vi "tcp client example.vi"() -> ()   [LabVIEW 2013]
doc: "# #############################################################################\n# ATTENTION\n# #############################################################################\n#\n# This software is for guidance only. It is provided \"as is\".\n# It only aims at providing coding information to the customer in order for\n# them to save time. As a result no warranties, whether express, implied or\n# statutory, including, but not limited to implied warranties of\n# merchantability and fitness for a particular purpose apply to this software.\n# A·P·E Angewandte Physik und Elektronik GmbH shall not be held liable for any\n# direct, indirect or consequential damages with respect to any claims arising\n# from the content of such sourcecode and/or the use made by customers of the\n# coding information contained herein in connection with their products.\n#\n# #############################################################################"
uses:
  queue control/queue cluster.ctl
  <vilib>/Utility/miscctls.llb/LVPointTypeDef.ctl
panel:
  out "STOP":bool=TRUE
  out "error out":errorcluster
  out "Answer":string
  in  "Send":bool
  in  "CMD":string="*idn?\n" caption="Command"
  in  "Connect":bool
  in  "IP":string="127.0.0.1" caption="IP / Hostname"
  in  "PORT":u16=51019 caption="TCP Port"
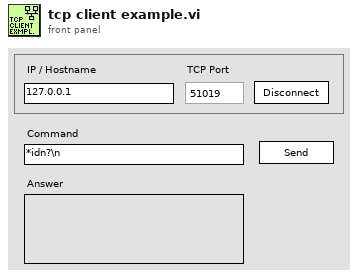
[diagram p1: front panel]
types:
  T1 = typedef "queue cluster.ctl" = cluster{"command":string, "data":variant}
  T2 = typedef "LVPointTypeDef.ctl" = cluster{"Horizontal":i16, "Vertical":i16}
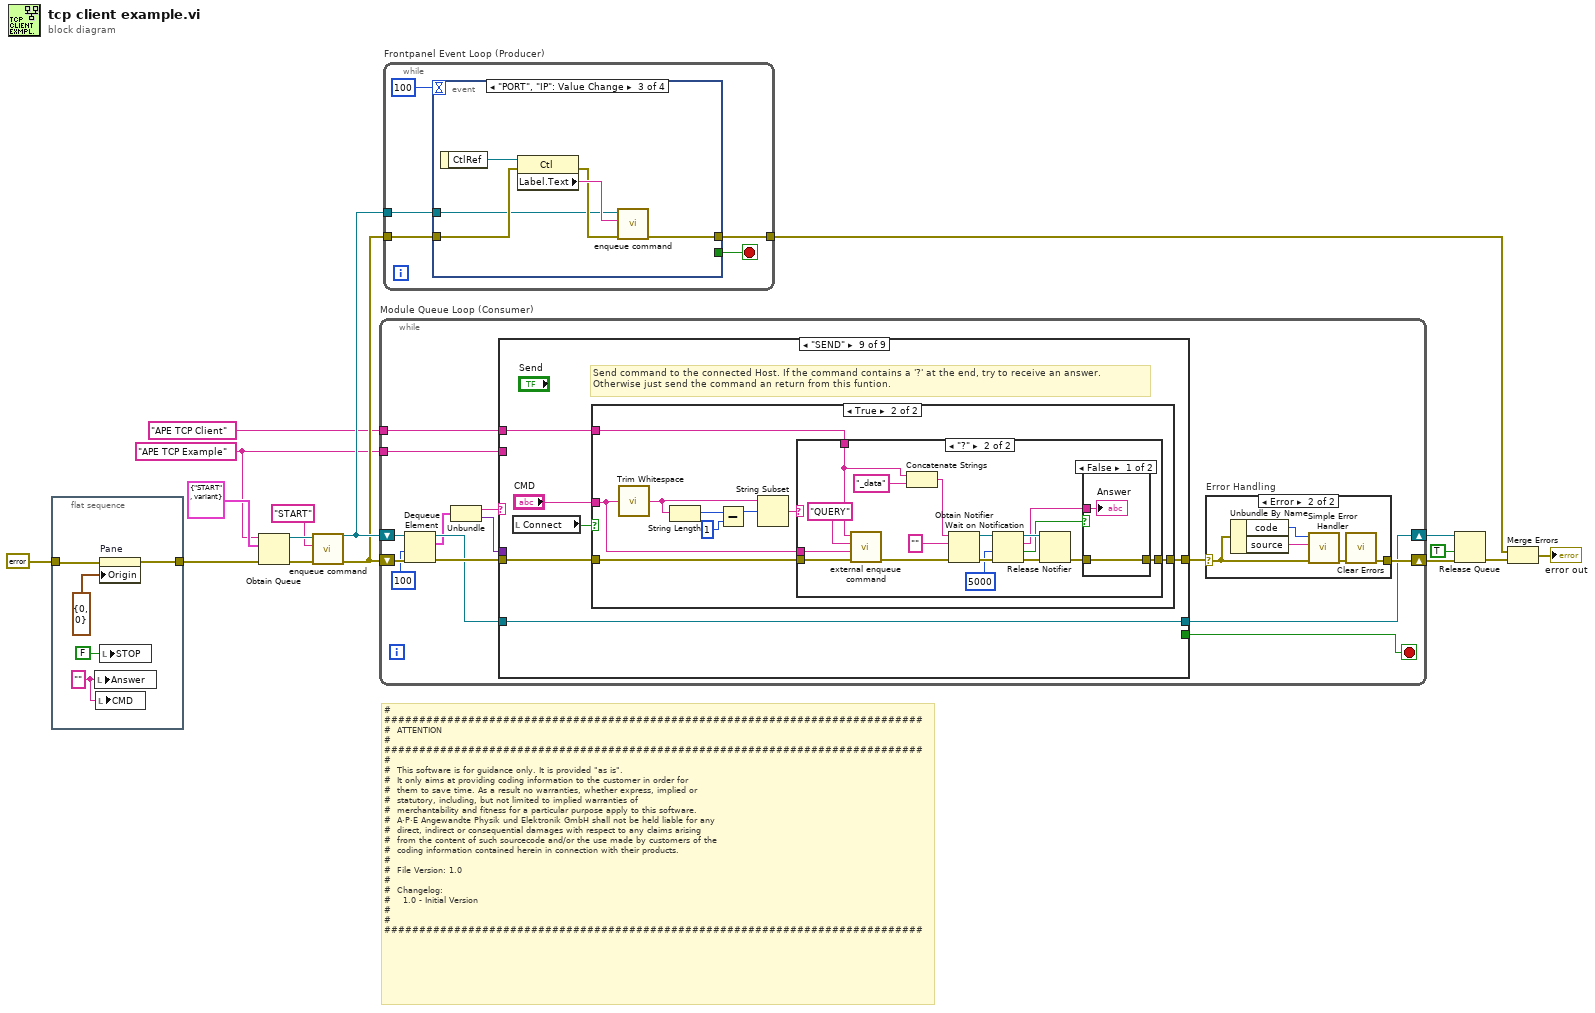
[diagram p0: block diagram]
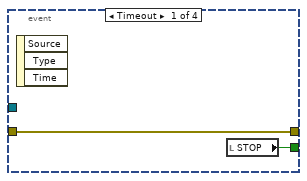
[diagram p2: hidden frame]
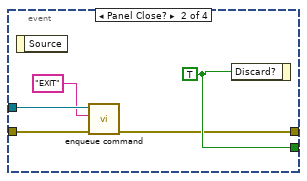
[diagram p3: hidden frame]
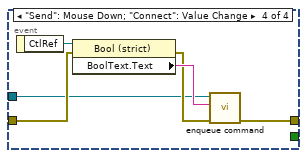
[diagram p4: hidden frame]
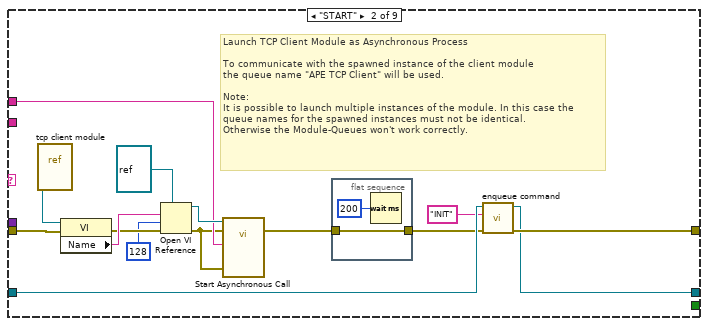
[diagram p7: hidden frame]
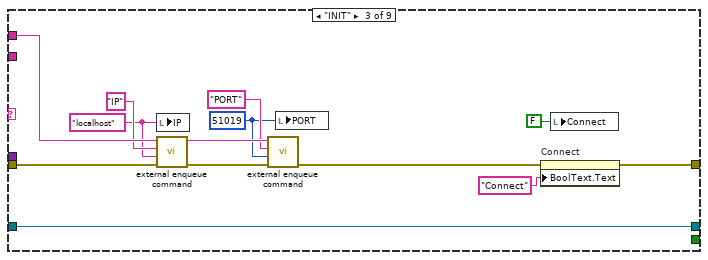
[diagram p8: hidden frame]
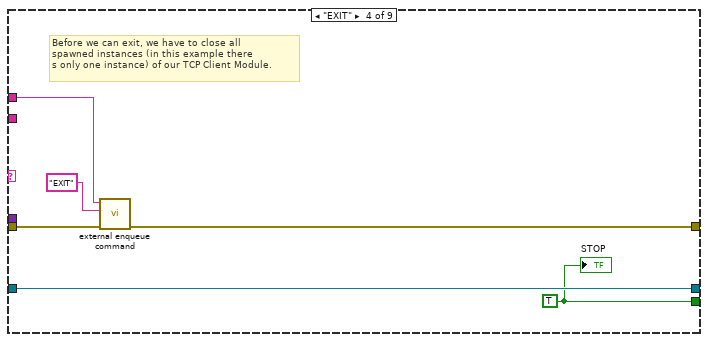
[diagram p9: hidden frame]
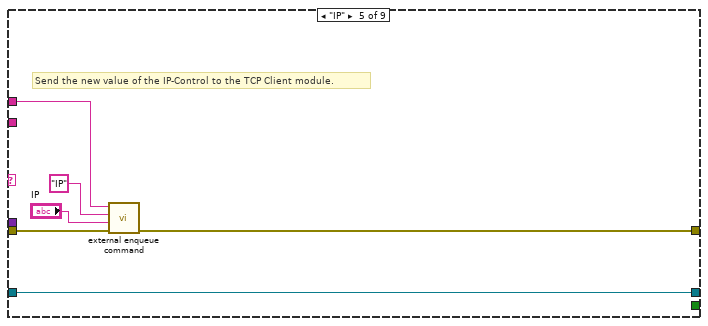
[diagram p10: hidden frame]
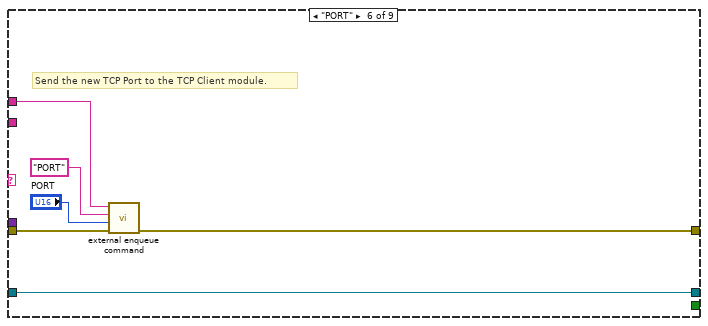
[diagram p11: hidden frame]
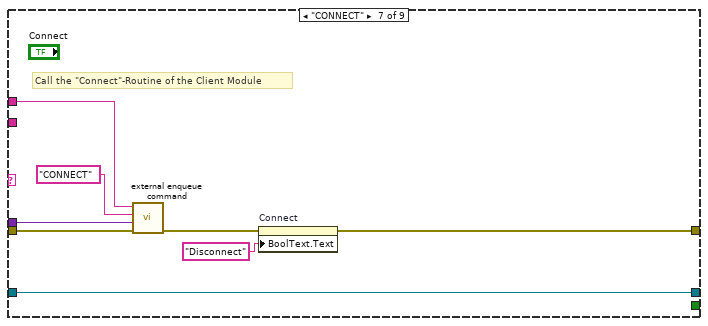
[diagram p12: hidden frame]
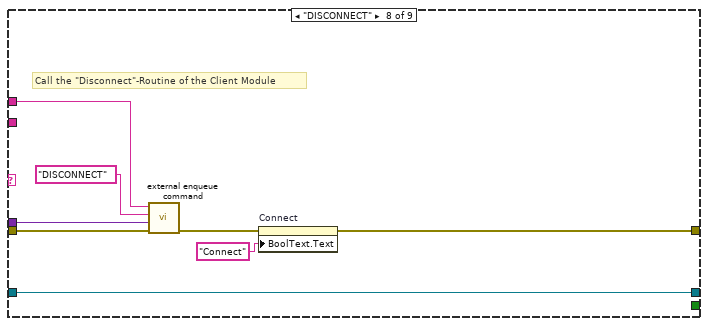
[diagram p13: hidden frame]
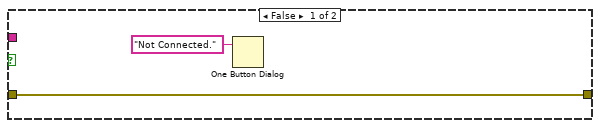
[diagram p14: hidden frame]
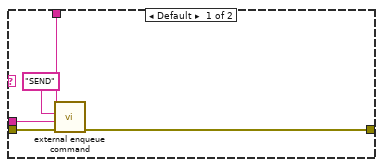
[diagram p15: hidden frame]
diagram:
  w1 = "APE TCP Example" ("name (unnamed)")
  # "# #############################################################################\n#  ATTENTION\n# #############################################################################\n#\n#  This software is for guidance only. It is provided \"as is\".\n#  It only aims at providing coding information to the customer in order for\n#  them to save time. As a result no warranties, whether express, implied or\n#  statutory, including, but not limited to implied warranties of\n#  merchantability and fitness for a particular purpose apply to this software.\n#  A·P·E Angewandte Physik und Elektronik GmbH shall not be held liable for any\n#  direct, indirect or consequential damages with respect to any claims arising\n#  from the content of such sourcecode and/or the use made by customers of the\n#  coding information contained herein in connection with their products.\n#\n#  File Version: 1.0\n#\n#  Changelog:\n#    1.0 - Initial Version\n#\n# #############################################################################"
  n1 = flat-sequence {
    tunnel: errorcluster {"status"=FALSE, "code"=0, "source"=""} ("error in (no error)") -> [w18]
    tunnel: [w20] -> w3
    frame #0 {
      w17 = "" ("Answer")
      n2 = local write "Answer"(w17) -> ()
      n3 = local write "CMD"(w17) -> ()
      n4 = property on="Pane" class="Pane"(error in=w18, "Origin"=T2 {"Horizontal"=0, "Vertical"=0}) -> (error out=w20:errorcluster)  [unwired: 1 in, 1 out]
      n5 = local write "STOP"(FALSE ("STOP")) -> ()
    }
  }
  n6 = Obtain Queue(name (unnamed)=w1, element data type=T1 {"command"="START", "data"=variant} ("QDSM"), error in (no error)=w3) -> (queue out=w14:refnum<queue>, error out=w15:errorcluster)  [unwired: 2 in, 1 out]
  n7 = call "enqueue command.vi"("error in"=w15, "Command"="START", "Queue in"=w14) -> ("error out"=w11:errorcluster, "Queue out"=w12:refnum<queue>)  [unwired: 7 in]
  n8 = while "Module Queue Loop (Consumer)" {
    shift-right: [w29] -> w7
    shift-left: w12 -> [w34]
    shift-right: [w31] -> w10
    shift-left: w11 -> [w35]
    tunnel: "APE TCP Client" ("name (unnamed)") -> [w23]
    tunnel: w1 -> [w22]
    stop <- w24 stop-if-true
    n9 = Dequeue Element(queue=w34, timeout in ms (-1)=100 ("timeout out"), error in (no error)=w35) -> (queue out=w32:refnum<queue>, element=w28:T1, error out=w33:errorcluster)  [unwired: 1 out]
    n10 = Unbundle(w28) -> ("command"=w27:string, "data"=w26:variant)
    n11 = case shown="\"SEND\"" w27 {
      tunnel: [w43 w49 w62 w76 w83 w89 w93 w101 w110] -> w30
      tunnel: w33 -> [w43 w53 w72 w77 w84 w90 w98 w106 w112]
      tunnel: [w42 w47 w73 w79 w85 w91 w99 w107 w113] -> w29
      tunnel: w32 -> [w42 w48 w73 w79 w85 w91 w99 w107 w113]
      tunnel: w26 -> [_ _ _ _ _ _ w95 w103 _]
      tunnel: [_ _ _ w78 _ _ _ _ _] -> w24
      tunnel: w23 -> [_ w51 w71 w75 w82 w88 w97 w105 w111]
      tunnel: w22 -> [_ _ _ _ _ _ _ _ _]
      frame Default {
        # "If you end up here, a Command was dequeued that is unknown to this case structure.\n\nYou may implement some kind of error-handlind or a user-message here, to become aware of this issue."
      }
      frame "START" {
        # "Launch TCP Client Module as Asynchronous Process\n\nTo communicate with the spawned instance of the client module\nthe queue name \"APE TCP Client\" will be used.\n\nNote:\nIt is possible to launch multiple instances of the module. In this case the \nqueue names for the spawned instances must not be identical.\nOtherwise the Module-Queues won't work correctly."
        n12 = vi-ref "tcp client module.vi"() -> (w56:refnum<vi>)
        n13 = property class="VI"(reference=w56, error in=w53) -> (error out=w57:errorcluster, "Name"=w58:string)  [unwired: 1 out]
        n14 = Open VI Reference(type specifier VI Refnum (for type only)=refnum<vi> refnum, vi path=w58, options=128, error in (no error)=w57) -> (vi reference=w54:refnum<vi>, error out=w50:errorcluster)  [unwired: 2 in]
        n15 = call-by-ref "Start Asynchronous Call"(reference=w54, error in=w50, "error in"=w50, "name"=w51) -> (error out=w44:errorcluster)  [unwired: 9 in, 2 out]
        n16 = flat-sequence {
          tunnel: [w60] -> w45
          tunnel: w44 -> [w60]
          frame #0 {
            n17 = Wait (ms)(milliseconds to wait=u32 200) -> ()  [unwired: 1 out]
          }
        }
        n18 = call "enqueue command.vi"("error in"=w45, "Command"="INIT", "Queue in"=w48) -> ("error out"=w49:errorcluster, "Queue out"=w47:refnum<queue>)  [unwired: 7 in]
      }
      frame "INIT" {
        w65 = u16 51019 ("timeout out")
        w66 = "localhost" ("Command")
        n19 = local write "IP"(w66) -> ()
        n20 = call "external enqueue command.vi"("error in"=w72, "Data"=w66, "Command"="IP", "Queuename"=w71) -> ("error out"=w70:errorcluster, "Queuename dup"=w69:string)  [unwired: 6 in]
        n21 = call "external enqueue command.vi"("error in"=w70, "Data"=w65, "Command"="PORT", "Queuename"=w69) -> ("error out"=w61:errorcluster)  [unwired: 6 in, 1 out]
        n22 = local write "PORT"(w65) -> ()
        n23 = property on="Connect" class="Bool (strict)"(error in=w61, "BoolText.Text"="Connect" ("Boolean Text.Text")) -> (error out=w62:errorcluster)  [unwired: 1 in, 1 out]
        n24 = local write "Connect"(FALSE ("Connect")) -> ()
      }
      frame "EXIT" {
        w78 = TRUE
        # "Before we can exit, we have to close all \nspawned instances (in this example there \ns only one instance) of our TCP Client Module."
        n25 = call "external enqueue command.vi"("error in"=w77, "Command"="EXIT", "Queuename"=w75) -> ("error out"=w76:errorcluster)  [unwired: 7 in, 1 out]
        "STOP" <- w78
      }
      frame "IP" {
        # "Send the new value of the IP-Control to the TCP Client module."
        n26 = call "external enqueue command.vi"("error in"=w84, "Data"="IP", "Command"="IP", "Queuename"=w82) -> ("error out"=w83:errorcluster)  [unwired: 6 in, 1 out]
      }
      frame "PORT" {
        # "Send the new TCP Port to the TCP Client module."
        n27 = call "external enqueue command.vi"("error in"=w90, "Data"="PORT", "Command"="PORT", "Queuename"=w88) -> ("error out"=w89:errorcluster)  [unwired: 6 in, 1 out]
      }
      frame "CONNECT" {
        # "Call the \"Connect\"-Routine of the Client Module"
        n28 = call "external enqueue command.vi"("error in"=w98, "Data"=w95, "Command"="CONNECT", "Queuename"=w97) -> ("error out"=w94:errorcluster)  [unwired: 6 in, 1 out]
        n29 = property on="Connect" class="Bool (strict)"(error in=w94, "BoolText.Text"="Disconnect" ("Boolean Text.Text")) -> (error out=w93:errorcluster)  [unwired: 1 in, 1 out]
      }
      frame "DISCONNECT" {
        # "Call the \"Disconnect\"-Routine of the Client Module"
        n30 = call "external enqueue command.vi"("error in"=w106, "Data"=w103, "Command"="DISCONNECT", "Queuename"=w105) -> ("error out"=w102:errorcluster)  [unwired: 6 in, 1 out]
        n31 = property on="Connect" class="Bool (strict)"(error in=w102, "BoolText.Text"="Connect" ("Boolean Text.Text")) -> (error out=w101:errorcluster)  [unwired: 1 in, 1 out]
      }
      frame "SEND" {
        # "Send command to the connected Host. If the command contains a '?' at the end, try to receive an answer.\nOtherwise just send the command an return from this funtion."
        n32 = local read "Connect"() -> (w109:bool)
        n33 = case shown="True" w109 {
          tunnel: w112 -> [w115 w124]
          tunnel: w111 -> [_ w123]
          tunnel: [w115 w122] -> w110
          tunnel: "CMD" -> [_ w117]
          frame False {
            n34 = One Button Dialog(message="Not Connected.") -> ()  [unwired: 1 in, 1 out]
          }
          frame True {
            n35 = call <vilib>:"Trim Whitespace.vi"("string"=w117) -> ("trimmed string"=w119:string)  [unwired: 1 in]
            n36 = String Length(string=w119) -> (length=w121:i32)
            n37 = Subtract(x=w121, y=1) -> (x-y=w120:i32)
            n38 = String Subset(string=w119, offset (0)=w120) -> (substring=w118:string)  [unwired: 1 in]
            n39 = case shown="\"?\"" w118 {
              tunnel: w124 -> [w128 w146]
              tunnel: w123 -> [w126 w130]
              tunnel: [w127 w135] -> w122
              tunnel: w117 -> [w125 w131]
              frame Default {
                n40 = call "external enqueue command.vi"("error in"=w128, "Data"=w125, "Command"="SEND", "Queuename"=w126) -> ("error out"=w127:errorcluster)  [unwired: 6 in, 1 out]
              }
              frame "?" {
                n41 = call "external enqueue command.vi"("error in"=w146, "Data"=w131, "Command"="QUERY", "Queuename"=w130) -> ("error out"=w139:errorcluster)  [unwired: 6 in, 1 out]
                n42 = Concatenate Strings(w130, "_data" ("string")) -> (w137:string)
                n43 = Obtain Notifier(name (unnamed)=w137, notification data type="", error in (no error)=w139) -> (notifier out=w143:refnum<notifier>, error out=w140:errorcluster)  [unwired: 1 in, 1 out]
                n44 = Wait on Notification(notifier=w143, timeout in ms (-1)=5000, error in (no error)=w140) -> (notifier out=w144:refnum<notifier>, notification=w132:string, timed out?=w133:bool, error out=w141:errorcluster)  [unwired: 1 in]
                n45 = Release Notifier(notifier=w144, error in (no error)=w141) -> (error out=w134:errorcluster)  [unwired: 1 in, 2 out]
                n46 = case shown="False" w133 {
                  tunnel: [w148 w149] -> w135
                  tunnel: w134 -> [w148 w149]
                  tunnel: w132 -> [w147 _]
                  frame False {
                    "Answer" <- w147
                  }
                  frame True {
                  }
                }
              }
            }
          }
        }
      }
    }
    n47 = case "Error Handling" shown="Error" w30 {
      selector: w30 -> [w36 w40]
      tunnel: [w36 w37] -> w31
      frame No Error {
      }
      frame Error {
        n48 = Unbundle By Name(w40) -> ("code"=w39:i32, "source"=w38:string)
        n49 = call <vilib>:"Simple Error Handler.vi"("error code (no error:0)"=w39, "error source (\" \")"=w38, "error in (no error)"=w40) -> ("error out"=w41:errorcluster)  [unwired: 2 in, 4 out]
        n50 = call <vilib>:"Clear Errors.vi"("error in (no error)"=w41) -> ("error out"=w37:errorcluster)  [unwired: 5 in, 1 out]
      }
    }
  }
  n51 = while "Frontpanel Event Loop (Producer)" {
    tunnel: w12 -> [w154]
    tunnel: w11 -> [w153]
    tunnel: [w151] -> w8
    stop <- w150 stop-if-true
    n52 = event shown="[2] \"PORT\", \"IP\": Value Change" {
      selector: _ -> [_ _ _ _]
      dyn-events: _ -> [_ _ _ _]
      timeout: 100 -> [_ _ _ _]
      tunnel: w154 -> [_ w158 w163 w169]
      tunnel: w153 -> [w156 w160 w167 w173]
      tunnel: [w156 w159 w162 w168] -> w151
      tunnel: [w155 w161 _ _] -> w150
      event Timeout {
        n53 = event-data() -> ()  [unwired: 1 in, 3 out]
        n54 = local read "STOP"() -> (w155:bool)
      }
      event Panel Close? {
        w161 = TRUE
        n55 = event-data() -> ()  [unwired: 1 in, 1 out]
        n56 = call "enqueue command.vi"("error in"=w160, "Command"="EXIT", "Queue in"=w158) -> ("error out"=w159:errorcluster)  [unwired: 7 in, 1 out]
        n57 = event-data("Discard?"=w161) -> ()  [unwired: 1 in, 1 out]
      }
      event "PORT", "IP": Value Change {
        n58 = event-data() -> ("CtlRef"=w166:refnum<vi>)  [unwired: 1 in]
        n59 = property class="Ctl"(reference=w166, error in=w167) -> (error out=w164:errorcluster, "Label.Text"=w165:string)  [unwired: 1 out]
        n60 = call "enqueue command.vi"("error in"=w164, "Command"=w165, "Queue in"=w163) -> ("error out"=w162:errorcluster)  [unwired: 7 in, 1 out]
      }
      event "Send": Mouse Down; "Connect": Value Change {
        n61 = event-data() -> ("CtlRef"=w172:refnum<vi>)  [unwired: 1 in]
        n62 = property class="Bool (strict)"(reference=w172, error in=w173) -> (error out=w170:errorcluster, "BoolText.Text"=w171:string)  [unwired: 1 out]
        n63 = call "enqueue command.vi"("error in"=w170, "Command"=w171, "Queue in"=w169) -> ("error out"=w168:errorcluster)  [unwired: 7 in, 1 out]
      }
    }
  }
  n64 = Release Queue(queue=w7, force destroy? (F)=TRUE, error in (no error)=w10) -> (error out=w9:errorcluster)  [unwired: 2 out]
  n65 = Merge Errors(w8, w9) -> (→"error out":errorcluster)
